vi "ControlPlansList.vi"(8 "error in (no error)":errorcluster, 11 "ByteGSAPIBase in":refnum<class "ByteGSAPIBase.lvclass">) -> (0 "error out":errorcluster, 2 "Control plans":T1[](array[typedef]), 3 "ByteGSAPIBase out":refnum<class "ByteGSAPIBase.lvclass">)   [LabVIEW 2019, in "ByteGSWebAPI.lvlib" / "ByteGSAPIBase.lvclass"]
uses:
  ByteGSAPIBase.lvclass
  ControlPlan.ctl
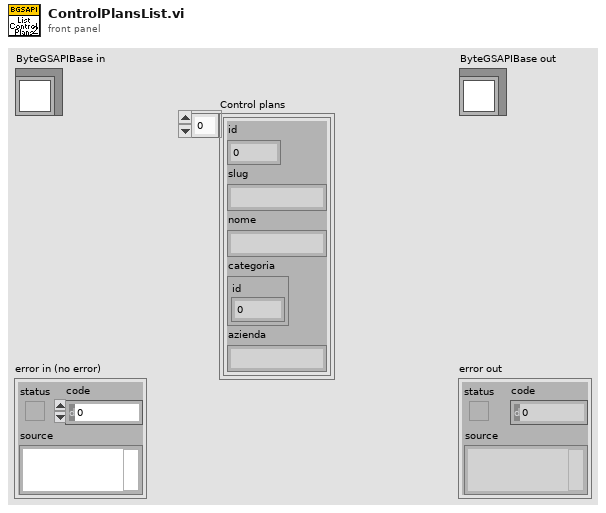
[diagram p1: front panel]
types:
  T1 = typedef "ByteGSWebAPI.lvlib/ByteGSAPIBase.lvclass/ControlPlan.ctl" = cluster{"id":i32, "slug":string, "nome":string, "categoria":cluster{"id":i32}, "azienda":string}
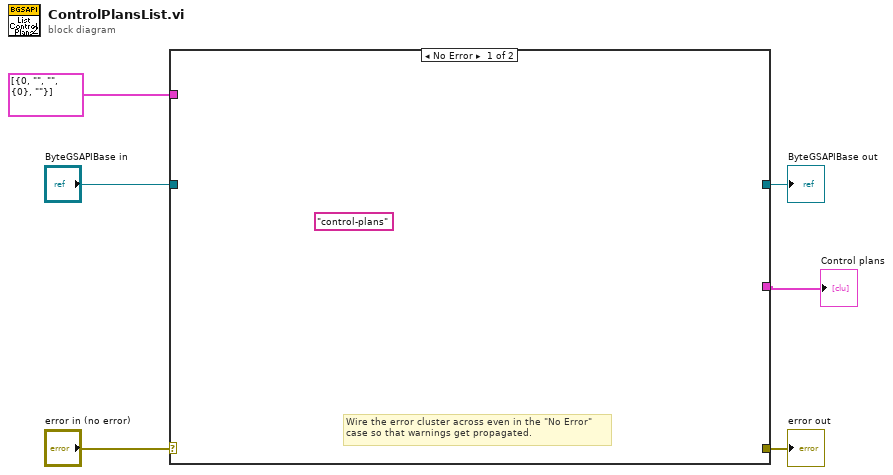
[diagram p0: block diagram]
diagram:
  n1 = case shown="No Error" "error in (no error)" {
    selector: "error in (no error)" -> [w10 w16]
    tunnel: [w9 w16] -> w5
    tunnel: [w12 w15] -> w3
    tunnel: "ByteGSAPIBase in" -> [w13 w15]
    tunnel: T1[] [{"id"=0, "slug"="", "nome"="", "categoria"={"id"=0}, "azienda"=""}] -> [w8 w14]
    tunnel: [w7 w14] -> w1
    frame No Error {
      w11 = "control-plans" ("Request")
      # "Wire the error cluster across even in the \"No Error\"\ncase so that warnings get propagated."
    }
    frame Error {
    }
  }
  "error out" <- w5
  "ByteGSAPIBase out" <- w3
  "Control plans" <- w1
